vi "Get Sciscan Scope Position.vi"(8 "error in":errorcluster, 11 "GFG Refnum":refnum<vi>) -> (0 "error out":errorcluster, 2 "Position [um]":T1, 3 "GFG Refnum Out":refnum<vi>)   [LabVIEW 2012, in "Sciscan Scope Daemon.lvlib"]
uses:
  Sciscan Scope Daemon.lvlib
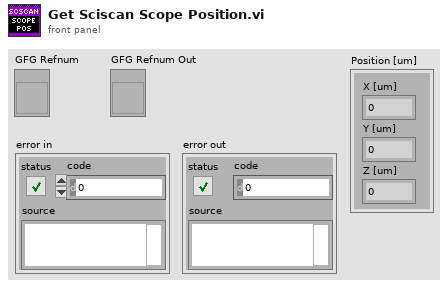
[diagram p1: front panel]
types:
  T1 = cluster{"X [um]":dbl, "Y [um]":dbl, "Z [um]":dbl}
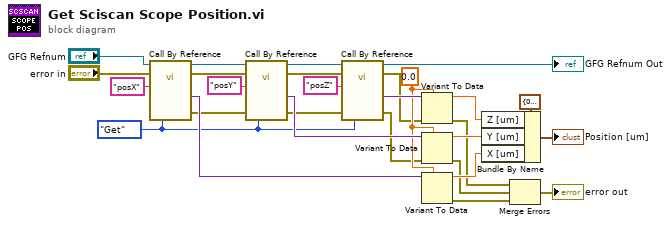
[diagram p0: block diagram]
diagram:
  w10 = 0.0
  w20 = enum16{"Init", "Set", "Get"}."Get" ("Action")
  n1 = call-by-ref "?"(reference="GFG Refnum", error in="error in", "Variable Name in"="posX", "Action"=w20) -> (reference out=w24:refnum<vi>, error out=w23:errorcluster, "Variant Out"=w27:variant, 19:"error out"=w16:errorcluster)  [unwired: 11 in, 5 out]
  n2 = call-by-ref "?"(reference=w24, error in=w23, "Variable Name in"="posY", 5:"error in (no error)"=w16, "Action"=w20) -> (reference out=w26:refnum<vi>, error out=w25:errorcluster, "Variant Out"=w22:variant, 19:"error out"=w15:errorcluster)  [unwired: 10 in, 5 out]
  n3 = call-by-ref "?"(reference=w26, error in=w25, "Variable Name in"="posZ", 5:"error in (no error)"=w15, "Action"=w20) -> (reference out=→"GFG Refnum Out":refnum<vi>, error out=w6:errorcluster, "Variant Out"=w21:variant, 19:"error out"=w5:errorcluster)  [unwired: 10 in, 5 out]
  n4 = Variant To Data(error in=w6, type=w10, Variant=w21) -> (data=w8:dbl, error out=w2:errorcluster)
  n5 = Variant To Data(error in=w5, type=w10, Variant=w22) -> (data=w9:dbl, error out=w3:errorcluster)
  n6 = Variant To Data(type=w10, Variant=w27) -> (data=w7:dbl, error out=w4:errorcluster)  [unwired: 1 in]
  n7 = Bundle By Name(cluster=T1 {"X [um]"=0.0, "Y [um]"=0.0, "Z [um]"=0.0}, "Z [um]"=w8, "Y [um]"=w9, "X [um]"=w7) -> (→"Position [um]":T1)
  n8 = Merge Errors(w2, w3, w4) -> (→"error out":errorcluster)
